vi "Listen Timeout.vi"(8 "error in (no error)":errorcluster, 11 "Announcing in":refnum<class "Announcing.lvclass">) -> (0 "error out":errorcluster, 3 "Announcing out":refnum<class "Announcing.lvclass">)   [LabVIEW 2013, in "Receiver.lvlib" / "Receiver Commands Using Processor.lvlib" / "Connect Command.lvlib" / "Announcing.lvclass"]
uses:
  Announcing.lvclass
  Connect Command.lvclass
  <vilib>/ActorFramework/Actor/Actor.lvclass/Actor.ctl
  <vilib>/ActorFramework/Message Enqueuer/Message Enqueuer.lvclass/Message Enqueuer.ctl
  Receiver Messages/Annouce Msg/Annouce Msg.lvclass/Annouce Msg.ctl
  <vilib>/ActorFramework/Message Enqueuer/Init from Existing Queue.vi
  <vilib>/ActorFramework/Message Enqueuer/Enqueue.vi
  <vilib>/ActorFramework/Message Priority Queue/Priority Enqueue.vi
  <vilib>/ActorFramework/Message Enqueuer/Message Enqueuer.lvclass
  Receiver Messages/Annouce Msg/Annouce Msg.lvclass
  <vilib>/ActorFramework/Actor/Actor.lvclass
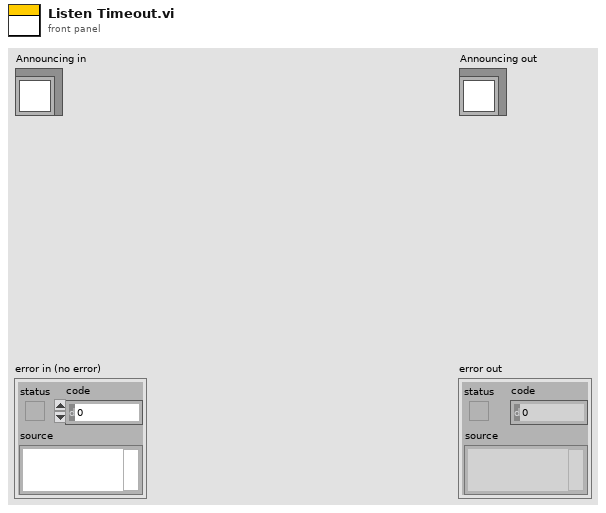
[diagram p1: front panel]
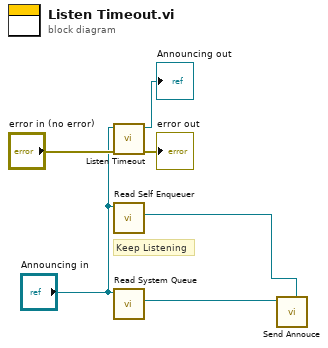
[diagram p0: block diagram]
diagram:
  # "Keep Listening"
  n1 = call-parent "Listen Timeout.vi"("error in (no error)"="error in (no error)", "Receiver Command in"="Announcing in") -> ("error out"=→"error out":errorcluster, "Receiver Command out"=→"Announcing out":refnum<class "Announcing.lvclass">)  [unwired: 8 in]
  n2 = call <vilib>:"Read Self Enqueuer.vi"("Actor"="Announcing in") -> ("Self Enqueuer"=w1:refnum<class "Message Enqueuer.lvclass">)  [unwired: 10 in]
  n3 = call-dynamic "Read System Queue.vi"("Command in"="Announcing in") -> ("Actor Framework:Message Enqueuer"=w2:refnum<class "Message Enqueuer.lvclass">)  [unwired: 8 in, 2 out]
  n4 = call "Send Annouce.vi"("Command Queue"=w1, "Message Enqueuer"=w2) -> ()  [unwired: 8 in, 2 out]
